vi "_Parse SEM Extreme Limit Check Result.vi"(8 "error in (no error)":errorcluster, 10 "Input String":string, 11 "VISA resource name":refnum<visa-resource-name>) -> (0 "error out":errorcluster, 1 "Measurement Result":T1 {"Out Of Tolerance" format="%^.3e"}, 2 "Reliability":i32, 3 "VISA resource name out":refnum<visa-resource-name>)   [LabVIEW 2020, in "Rohde&Schwarz CMXP NR FR2 Measurement.lvlib"]
uses:
  <instrlib>/Rohde&Schwarz CMXP NR FR2 Measurement/Rohde&Schwarz CMXP NR FR2 Measurement.lvlib
  <instrlib>/Rohde&Schwarz CMXP NR FR2 Measurement/Private/rsidr_core.llb/rsidr_core.lvlib
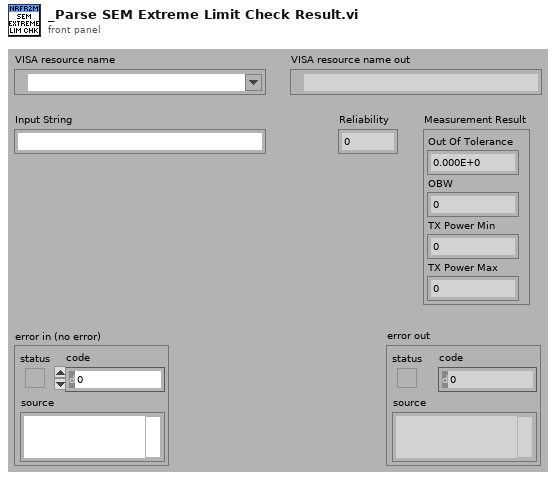
[diagram p1: front panel]
types:
  T1 = cluster{"Out Of Tolerance":dbl, "OBW":i32, "TX Power Min":i32, "TX Power Max":i32}
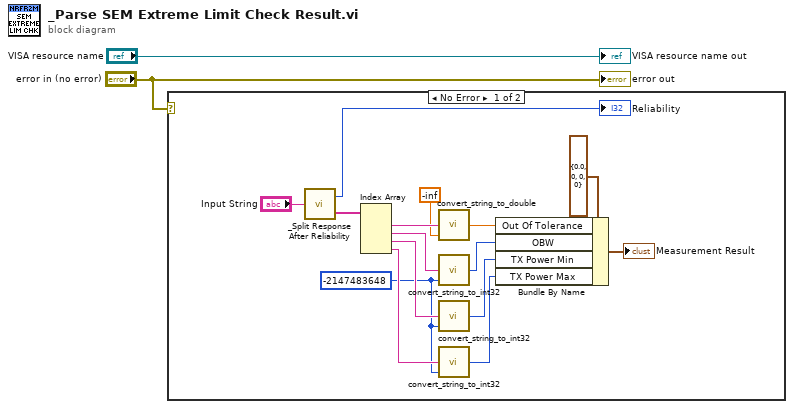
[diagram p0: block diagram]
diagram:
  n1 = case shown="No Error" "error in (no error)" {
    frame No Error {
      w5 = -2147483648
      n2 = call <instrlib>:"_Split Response After Reliability.vi"("Input String"="Input String") -> ("Response out"=w12:string[], "Reliability out"=→"Reliability":i32)
      n3 = Index Array(array=w12) -> (element #1=w11:string, element #2=w10:string, element #3=w9:string, element #4=w7:string)  [unwired: 4 in]
      n4 = call <instrlib>:"convert_string_to_double.vi"("default (0)"=-inf, "String in"=w11) -> ("double value out"=w17:dbl)  [unwired: 3 in]
      n5 = call <instrlib>:"convert_string_to_int32.vi"("default (0)"=w5, "String in"=w10) -> ("int32 value out"=w16:i32)  [unwired: 3 in]
      n6 = call <instrlib>:"convert_string_to_int32.vi"("default (0)"=w5, "String in"=w9) -> ("int32 value out"=w15:i32)  [unwired: 3 in]
      n7 = call <instrlib>:"convert_string_to_int32.vi"("default (0)"=w5, "String in"=w7) -> ("int32 value out"=w3:i32)  [unwired: 3 in]
      n8 = Bundle By Name(cluster=T1 {"Out Of Tolerance"=0.0, "OBW"=0, "TX Power Min"=0, "TX Power Max"=0} ("Measurement Result"), "Out Of Tolerance"=w17, "OBW"=w16, "TX Power Min"=w15, "TX Power Max"=w3) -> (→"Measurement Result":T1)
    }
    frame Error {
    }
  }
  "error out" <- "error in (no error)"
  "VISA resource name out" <- "VISA resource name"
